vi "PyArray_to_IMAQ.vi"(6 "Image Name":string="B_", 8 "error in (no error)":errorcluster, 10 "pythonArr_IN":u8[][][](array[numeric]), 11 "Refnum in":T1) -> (0 "error out":errorcluster, 2 "output size":i32[](array[numeric]), 3 "Refnum out":T1)   [LabVIEW 2021, in "Framework_lib.lvlib"]
uses:
  SubVis/QMH/Framework_lib.lvlib
  <vilib>/vision/Image Controls.llb/IMAQ Image.ctl
  <vilib>/vision/NI_Vision_Development_Module.lvlib
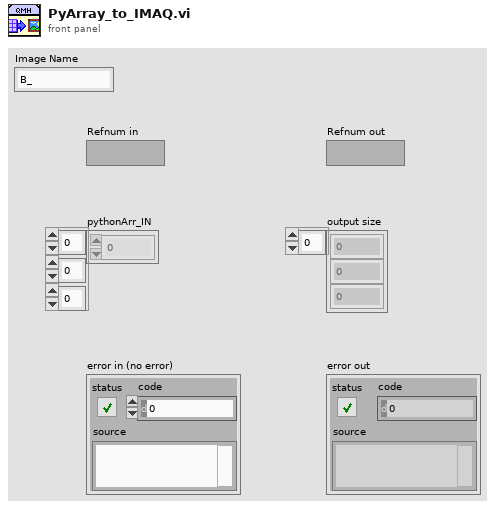
[diagram p1: front panel]
types:
  T1 = typedef "IMAQ Image.ctl" = refnum<image>
  T2 = typedef "Image Type" = u32
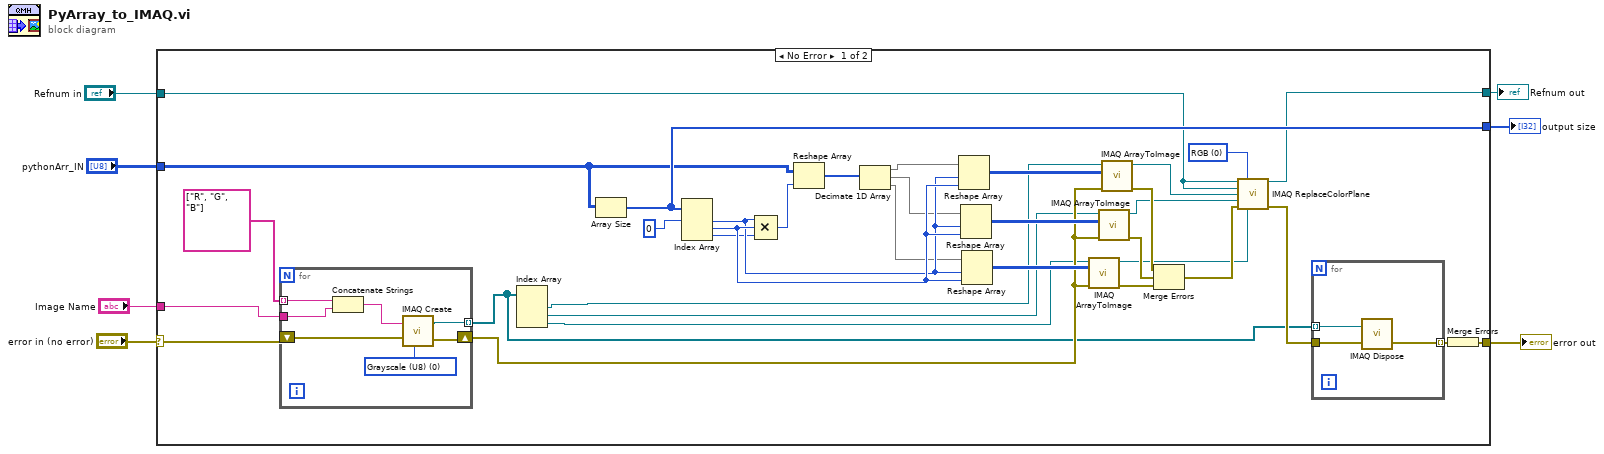
[diagram p0: block diagram]
diagram:
  n1 = case shown="No Error" "error in (no error)" {
    selector: "error in (no error)" -> [w18 w54]
    tunnel: [w22 _] -> w7
    tunnel: [w21 w53] -> w6
    tunnel: [w9 w54] -> w5
    tunnel: "Refnum in" -> [w20 w53]
    tunnel: "pythonArr_IN" -> [w19 _]
    tunnel: "Image Name" -> [w12 _]
    frame No Error {
      w33 = u16 0 items=["RGB", "HSL", "HSV", "HSI"] ("Color Mode")
      n2 = for {
        shift-right: [w50] -> w17
        shift-left: w18 -> [w51]
        tunnel: [w49] -> w8 mode=indexing
        tunnel: string[] ["R", "G", "B"] ("Image Name 2") -> [w48] mode=indexing
        tunnel: w12 -> [w46]
        w52 = T2 0 items=["Grayscale (U8)", "Grayscale (I16)", "Grayscale (SGL)", "Complex (CSG)", "RGB (U32)", "HSL (U32)", "RGB (U64)", "Grayscale (U16)"] ("Image Type")
        n3 = Concatenate Strings(w48, w46) -> (w47:string)
        n4 = call "IMAQ Create"("Image Name"=w47, "Image Type"=w52, "error in (no error)"=w51) -> ("New Image"=w49:T1, "error out"=w50:errorcluster)  [unwired: 2 in]
      }
      n5 = Index Array(array=w8) -> (element #1=w16:T1, element #2=w15:T1, element #3=w14:T1)  [unwired: 3 in]
      n6 = Array Size(array=w19) -> (size(s)=w22:i32[])
      n7 = Index Array(array=w22, index #1=0 ("index")) -> (element #1=w36:i32, element #2=w37:i32, element #3=w35:i32)  [unwired: 2 in]
      n8 = Compound Arithmetic op=MULTIPLY(w36, w37, w35) -> (w24:i32)
      n9 = Reshape Array(w19, w24) -> (w25:u8[])
      n10 = Decimate 1D Array(w25) -> (w26:u8[], w27:u8[], w28:u8[])
      n11 = Reshape Array(w26, w36, w37) -> (w29:u8[][])
      n12 = Reshape Array(w27, w36, w37) -> (w30:u8[][])
      n13 = Reshape Array(w28, w36, w37) -> (w39:u8[][])
      n14 = call "IMAQ ArrayToImage"("error in (no error)"=w17, "Image Pixels (U8)"=w39, "Image"=w14) -> ("error out"=w34:errorcluster, "Image Out"=w38:T1)  [unwired: 7 in]
      n15 = call "IMAQ ArrayToImage"("error in (no error)"=w17, "Image Pixels (U8)"=w30, "Image"=w15) -> ("error out"=w41:errorcluster, "Image Out"=w32:T1)  [unwired: 7 in]
      n16 = call "IMAQ ArrayToImage"("error in (no error)"=w17, "Image Pixels (U8)"=w29, "Image"=w16) -> ("error out"=w42:errorcluster, "Image Out"=w31:T1)  [unwired: 7 in]
      n17 = Merge Errors(w42, w41, w34) -> (w40:errorcluster)
      n18 = call "IMAQ ReplaceColorPlane"("Image Src"=w20, "Color Mode"=w33, "Image Dst"=w20, "Red or Hue Plane"=w31, "Green or Sat Plane"=w32, "error in (no error)"=w40, "Blue or Luma or Val or Inten Plane"=w38) -> ("Image Dst Out"=w21:T1, "error out"=w10:errorcluster)  [unwired: 7 in]
      n19 = for {
        tunnel: [w44] -> w11 mode=indexing
        tunnel: w10 -> [w45]
        tunnel: w8 -> [w43] mode=indexing
        n20 = call "IMAQ Dispose"("Image"=w43, "error in (no error)"=w45) -> ("error out"=w44:errorcluster)  [unwired: 4 in]
      }
      n21 = Merge Errors(w11) -> (w9:errorcluster)
    }
    frame Error {
    }
  }
  "output size" <- w7
  "Refnum out" <- w6
  "error out" <- w5
